vi "Save Image.vi"(5 "Path":string="C:\\Tmp", 6 "SN":string, 7 "Image Quality":u32=750, 8 "error in (no error)":errorcluster, 9 "PassFail":bool, 10 "Image Saved":T1(ring), 11 "Image":T2) -> (0 "error out":errorcluster)   [LabVIEW 2018]
uses:
  <vilib>/vision/Image Controls.llb/IMAQ Image.ctl
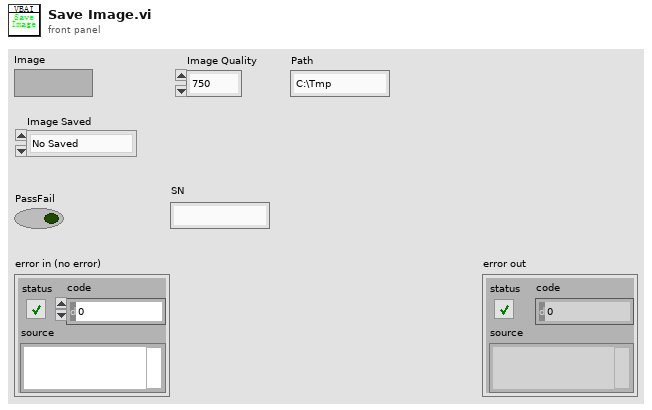
[diagram p1: front panel]
types:
  T1 = enum16{"No Saved", "All Saved", "Only Fail Saved"}
  T2 = typedef "IMAQ Image.ctl" = refnum<image>
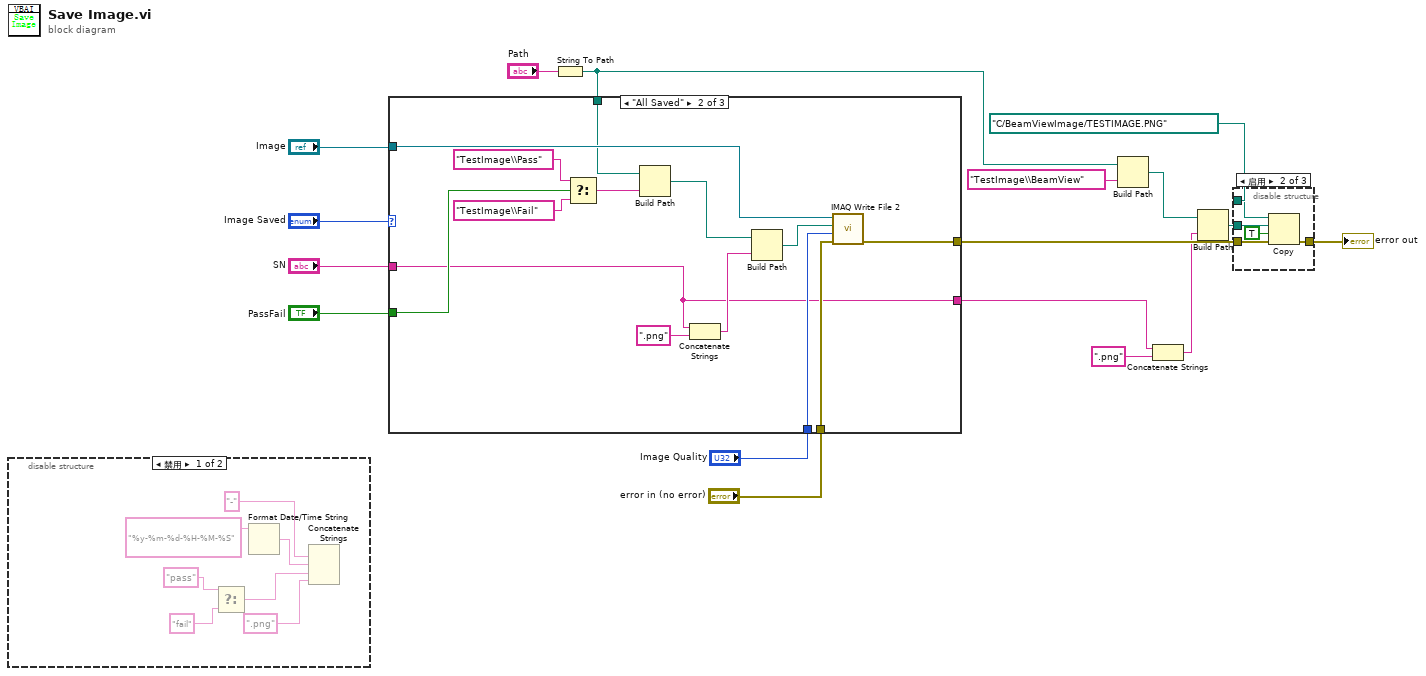
[diagram p0: block diagram]
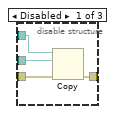
[diagram p3: hidden frame]
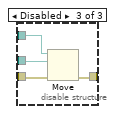
[diagram p4: hidden frame]
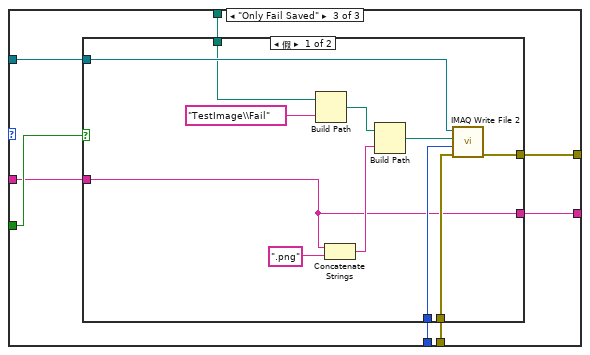
[diagram p6: hidden frame]
diagram:
  n1 = disable-structure shown="禁用" {
    frame Disabled {
      n2 = Select(t="pass" ("string"), f="fail") -> (s=w20:bool, s? t:f=w21:string)
      n3 = Format Date/Time String(time format string (%c)="%y-%m-%d-%H-%M-%S") -> (date/time string=w24:string)  [unwired: 2 in]
      n4 = Concatenate Strings("-", w24, w21, ".png" ("string")) -> (w18:string)  [unwired: 1 out]
    }
    frame Enabled {
    }
  }
  n5 = String To Path(string="Path") -> (path=w4:path)
  n6 = case shown="\"All Saved\"" "Image Saved" {
    tunnel: "Image" -> [_ w39 w50]
    tunnel: "PassFail" -> [_ w35 w47]
    tunnel: "error in (no error)" -> [w28 w33 w49]
    tunnel: [w28 w32 w48] -> w12
    tunnel: "Image Quality" -> [_ w31 w46]
    tunnel: w4 -> [_ w30 w45]
    tunnel: "SN" -> [w27 w29 w44]
    tunnel: [w27 w29 w43] -> w1
    frame "No Saved", Default {
    }
    frame "All Saved" {
      n7 = Select(t="TestImage\\Pass", s=w35, f="TestImage\\Fail") -> (s? t:f=w38:string)
      n8 = Build Path(base path=w30, name or relative path=w38) -> (appended path=w34:path)
      n9 = Concatenate Strings(w29, ".png" ("string")) -> (w41:string)
      n10 = Build Path(base path=w34, name or relative path=w41) -> (appended path=w40:path)
      n11 = call-poly "IMAQ Write File 2"("error in (no error)"=w33, "Image Quality"=w31, "File Path"=w40, "Image"=w39) -> ("error out"=w32:errorcluster)  [unwired: 6 in, 1 out]
    }
    frame "Only Fail Saved" {
      n12 = case shown="假" w47 {
        tunnel: w50 -> [w56 _]
        tunnel: w49 -> [w55 w63]
        tunnel: [w54 w63] -> w48
        tunnel: w46 -> [w53 _]
        tunnel: w45 -> [w52 _]
        tunnel: w44 -> [w51 w62]
        tunnel: [w51 w62] -> w43
        frame False {
          n13 = Build Path(base path=w52, name or relative path="TestImage\\Fail") -> (appended path=w58:path)
          n14 = Concatenate Strings(w51, ".png" ("string")) -> (w60:string)
          n15 = Build Path(base path=w58, name or relative path=w60) -> (appended path=w59:path)
          n16 = call-poly "IMAQ Write File 2"("error in (no error)"=w55, "Image Quality"=w53, "File Path"=w59, "Image"=w56) -> ("error out"=w54:errorcluster)  [unwired: 6 in, 1 out]
        }
        frame True {
        }
      }
    }
  }
  n17 = Build Path(base path=w4, name or relative path="TestImage\\BeamView") -> (appended path=w8:path)
  n18 = Concatenate Strings(w1, ".png" ("string")) -> (w5:string)
  n19 = Build Path(base path=w8, name or relative path=w5) -> (appended path=w7:path)
  n20 = disable-structure shown="启用" {
    disable-tunnel: w12 -> [w67 w72 w75]
    disable-tunnel: [w66 w71 w76] -> w11
    disable-tunnel: path "C:/BeamViewImage/TESTIMAGE.PNG" -> [w65 w70 w73]
    disable-tunnel: w7 -> [w64 w69 w74]
    frame Disabled {
      n21 = Copy(8:w67, 10:w64, 11:w65) -> (0:w66:errorcluster)  [unwired: 2 in, 2 out]
    }
    frame Enabled {
      n22 = Copy(8:w72, 9:TRUE ("覆盖(F)"), 10:w69, 11:w70) -> (0:w71:errorcluster)  [unwired: 1 in, 2 out]
    }
    frame Disabled {
      n23 = Move(source path=w73, error in=w75, 10:w74) -> (error out=w76:errorcluster)  [unwired: 2 in, 2 out]
    }
  }
  "error out" <- w11
